vi "Set Config Properties.vi"(8 "error in (no error)":errorcluster, 11 "WaveformCalculation in":refnum<class "WaveformCalculation.lvclass">) -> (0 "error out":errorcluster, 3 "WaveformCalculation out":refnum<class "WaveformCalculation.lvclass">)   [LabVIEW 2015, in "WaveformCalculation.lvclass"]
uses:
  Waveform-Processing-Custom-Device Configuration.llb/WaveformCalculation.lvclass
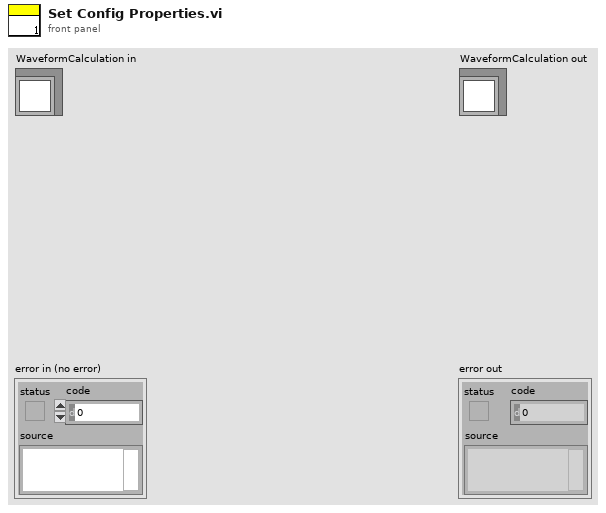
[diagram p1: front panel]
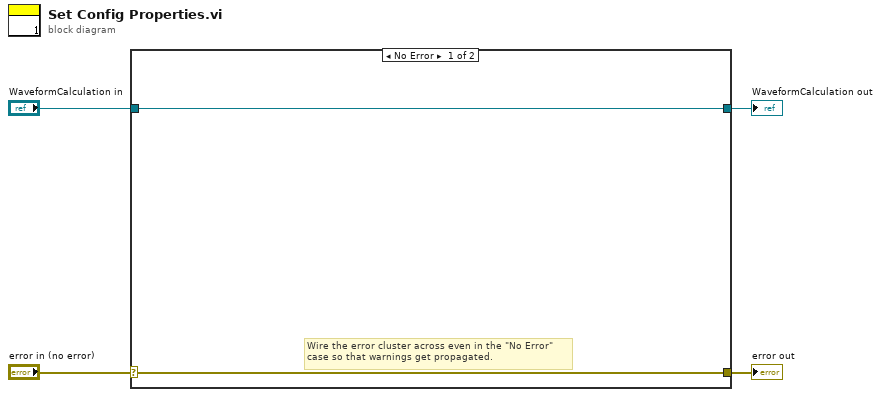
[diagram p0: block diagram]
diagram:
  n1 = case shown="No Error" "error in (no error)" {
    selector: "error in (no error)" -> [w6 w8]
    tunnel: [w6 w8] -> w3
    tunnel: [w5 w7] -> w1
    tunnel: "WaveformCalculation in" -> [w5 w7]
    frame No Error {
      # "Wire the error cluster across even in the \"No Error\"\ncase so that warnings get propagated."
    }
    frame Error {
    }
  }
  "error out" <- w3
  "WaveformCalculation out" <- w1
